vi "WPI_DashboardSeek to Scrub Time2.vi"(6 "Docked Window":bool, 7 "Version":i32=2, 8 "VI Refnum":refnum<vi>, 9 "latest update tick":timestamp, 10 "TimeOffset (s)":dbl, 11 "Byte Stream File in":refnum<file>) -> (0 "Strings":T1, 1 "ms tick out":timestamp, 2 "TimeOffset (s) out":dbl, 3 "Byte Stream File out":refnum<file>)   [LabVIEW 2025]
uses:
  <vilib>/Rock Robotics/WPI/Dashboard/WPI_DashboardNTL Header Type.ctl
  <vilib>/Rock Robotics/WPI/Dashboard/WPI_DashboardPlay Operation.ctl
  <vilib>/Rock Robotics/WPI/Dashboard/WPI_DashboardLogging Global.vi
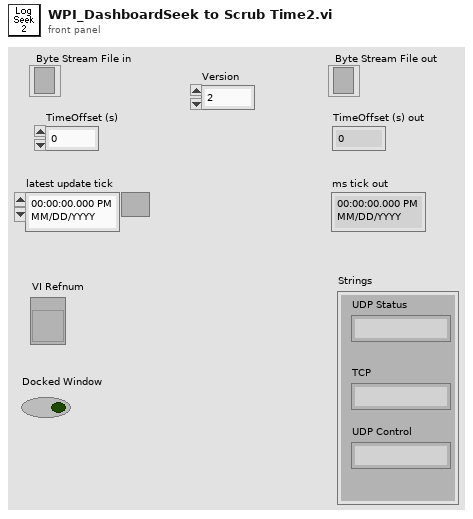
[diagram p1: front panel]
types:
  T1 = cluster{"UDP Status":string, "TCP":string, "UDP Control":string}
  T2 = typedef "WPI_DashboardPlay Operation.ctl" = enum16{"Play", "Pause", "Finished"}
  T3 = typedef "WPI_DashboardNTL Header Type.ctl" = cluster{"Version":i32, "Duration (ms)":i32, "TimeStamp":timestamp, "Robot IP":string, "Displays":string[]}
  T4 = enum16{"1/10", "1/5", "1/2", "1", "2", "5", "10"}
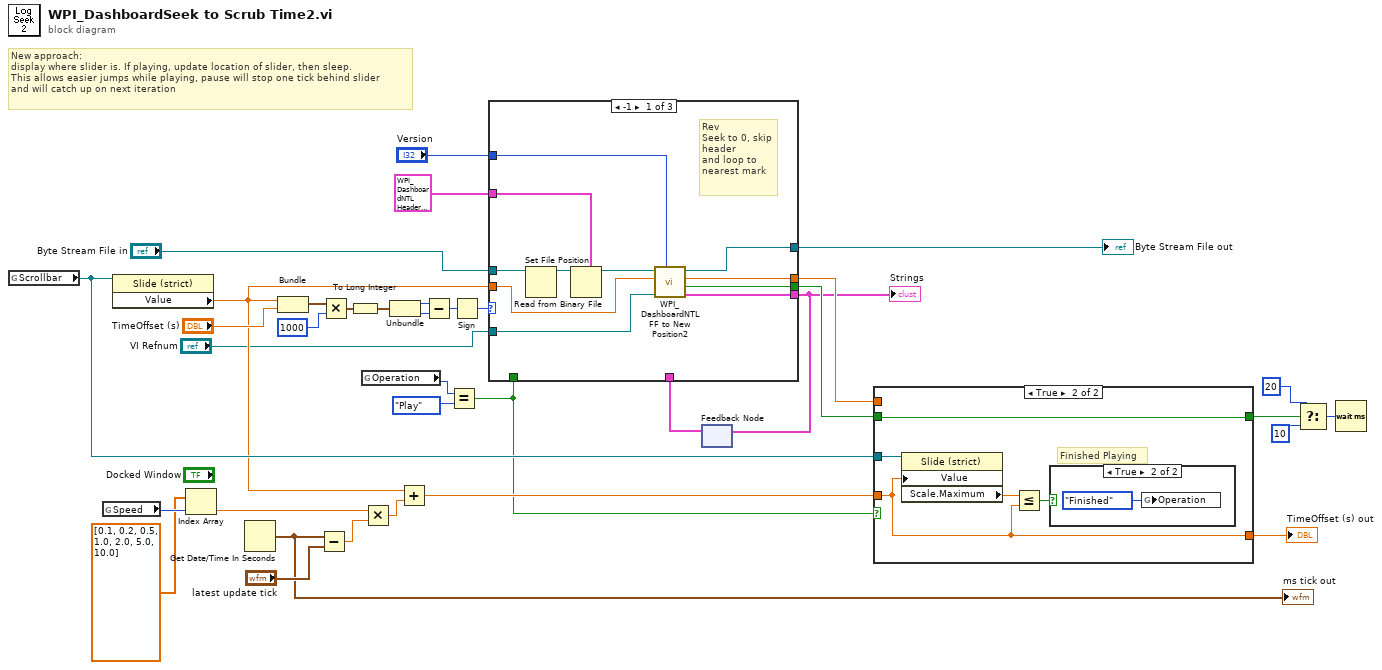
[diagram p0: block diagram]
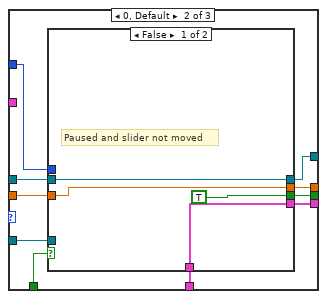
[diagram p4: hidden frame]
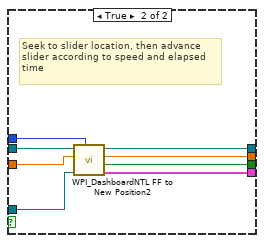
[diagram p5: hidden frame]
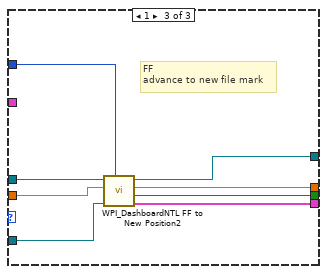
[diagram p6: hidden frame]
diagram:
  # "New approach:\ndisplay where slider is. If playing, update location of slider, then sleep.\nThis allows easier jumps while playing, pause will stop one tick behind slider\nand will catch up on next iteration"
  n1 = global read "WPI_DashboardLogging Global.vi" "Scrollbar"() -> (w17:refnum<vi>)
  n2 = global read "WPI_DashboardLogging Global.vi" "Speed"() -> (w31:T4)
  n3 = property class="Slide (strict)"(reference=w17) -> ("Value"=w5:dbl)  [unwired: 1 in, 2 out]
  n4 = Index Array(array=dbl[] [0.1, 0.2, 0.5, 1.0, 2.0, 5.0, 10.0], index=w31) -> (element=w29:dbl)
  n5 = Get Date/Time In Seconds() -> (seconds since 1Jan1904=w8:timestamp)
  "ms tick out" <- w8
  n6 = Bundle("Value"=w5, "TimeOffset (s)"="TimeOffset (s)") -> (w21:cluster{"Value":dbl, "TimeOffset (s)":dbl})  [unwired: 1 in]
  n7 = Subtract(x=w8, y="latest update tick") -> (x-y=w28:dbl)
  n8 = Multiply(x=w21, y=1000) -> (x*y=w22:cluster{"Value":dbl, "TimeOffset (s)":dbl})
  n9 = To Long Integer(number=w22) -> (32bit integer=w20:cluster{"Value":i32, "TimeOffset (s)":i32})
  n10 = global read "WPI_DashboardLogging Global.vi" "Operation"() -> (w18:T2)
  n11 = Multiply(x=w29, y=w28) -> (x*y=w16:dbl)
  n12 = Unbundle(w20) -> ("Value"=w24:i32, "TimeOffset (s)"=w23:i32)
  n13 = Add(x=w5, y=w16) -> (x+y=w13:dbl)
  n14 = Subtract(x=w24, y=w23) -> (x-y=w33:i32)
  n15 = Equal?(x=w18, y=WPI_DashboardPlay_Operation."Play" ("Operation")) -> (x = y?=w9:bool)
  n16 = Sign(1:w33) -> (0:w34:i32)
  n17 = feedback #1() -> (w4:T1)  [unwired: 1 in]
  n18 = case shown="-1" w34 {
    tunnel: "Byte Stream File in" -> [w47 w57 w77]
    tunnel: [w42 w56 w75] -> w36
    tunnel: T3 {"Version"=0, "Duration (ms)"=0, "TimeStamp"=timestamp(0 s since 1904-01-01), "Robot IP"="", "Displays"=[]} ("Header") -> [w45 _ _]
    tunnel: w5 -> [w38 w53 w76]
    tunnel: [w41 w55 w74] -> w15
    tunnel: [w43 w54 w73] -> w11
    tunnel: w9 -> [_ w52 _]
    tunnel: [w44 w51 w71] -> w2
    tunnel: w4 -> [_ w50 _]
    tunnel: "VI Refnum" -> [w39 w49 w72]
    tunnel: "Version" -> [w37 w48 w70]
    frame -1 {
      # "Rev\nSeek to 0, skip\nheader\nand loop to\nnearest mark"
      n19 = Set File Position(refnum=w47) -> (refnum out=w46:refnum<file>)  [unwired: 3 in, 1 out]
      n20 = Read from Binary File(5:w45, 11:w46) -> (3:w40:refnum<file>)  [unwired: 4 in, 3 out]
      n21 = call <vilib>:"WPI_DashboardNTL FF to New Position2.vi"("Version"=w37, "VI Refnum"=w39, "TimeOffset (s)"=w38, "Byte Stream File in"=w40) -> ("Strings"=w44:T1, "Unchanged"=w43:bool, "New time (s)"=w41:dbl, "Byte Stream File out"=w42:refnum<file>)  [unwired: 4 in]
    }
    frame 0, Default {
      n22 = case shown="False" w52 {
        tunnel: w57 -> [w61 w69]
        tunnel: [w61 w66] -> w56
        tunnel: [w59 w65] -> w55
        tunnel: [TRUE w64] -> w54
        tunnel: w53 -> [w59 w68]
        tunnel: [w58 w63] -> w51
        tunnel: w50 -> [w58 _]
        tunnel: w49 -> [_ w67]
        tunnel: w48 -> [_ w62]
        frame False {
          # "Paused and slider not moved"
        }
        frame True {
          # "Seek to slider location, then advance\nslider according to speed and elapsed\ntime"
          n23 = call <vilib>:"WPI_DashboardNTL FF to New Position2.vi"("Version"=w62, "VI Refnum"=w67, "TimeOffset (s)"=w68, "Byte Stream File in"=w69) -> ("Strings"=w63:T1, "Unchanged"=w64:bool, "New time (s)"=w65:dbl, "Byte Stream File out"=w66:refnum<file>)  [unwired: 4 in]
        }
      }
    }
    frame 1 {
      # "FF\nadvance to new file mark"
      n24 = call <vilib>:"WPI_DashboardNTL FF to New Position2.vi"("Version"=w70, "VI Refnum"=w72, "TimeOffset (s)"=w76, "Byte Stream File in"=w77) -> ("Strings"=w71:T1, "Unchanged"=w73:bool, "New time (s)"=w74:dbl, "Byte Stream File out"=w75:refnum<file>)  [unwired: 4 in]
    }
  }
  "Byte Stream File out" <- w36
  "Strings" <- w2
  n25 = feedback-in #1(w2) -> ()
  n26 = case shown="True" w9 {
    tunnel: w17 -> [_ w84]
    tunnel: w15 -> [w79 _]
    tunnel: w13 -> [_ w81]
    tunnel: [w79 w81] -> w14
    tunnel: [w78 w83] -> w10
    tunnel: w11 -> [w78 w83]
    frame False {
    }
    frame True {
      # "Finished Playing"
      n27 = property class="Slide (strict)"(reference=w84, "Value"=w81) -> ("Scale.Maximum"=w82:dbl)  [unwired: 1 in, 2 out]
      n28 = Less Or Equal?(x=w82, y=w81) -> (x <= y?=w80:bool)
      n29 = case shown="True" w80 {
        frame False {
        }
        frame True {
          n30 = global write "WPI_DashboardLogging Global.vi" "Operation"(WPI_DashboardPlay_Operation."Finished" ("Operation")) -> ()
        }
      }
    }
  }
  "TimeOffset (s) out" <- w14
  n31 = Select(t=20, s=w10, f=10) -> (s? t:f=w27:i32)
  n32 = Wait (ms)(milliseconds to wait=w27) -> ()  [unwired: 1 out]
